vi "Solve1.vi"(8 "Error In":errorcluster, 11 "object in":refnum<class "2022_6.lvclass">) -> (0 "Error Out":errorcluster, 2 "Result":u64, 3 "object out":refnum<class "2022_6.lvclass">)   [LabVIEW 2020, in "2022_6.lvclass"]
uses:
  2022_6.lvclass
  2022_6.lvclass/2022_6.ctl
  5bf5dcff-f428-4ee2-9bdf-71b01ce05b8f.vi
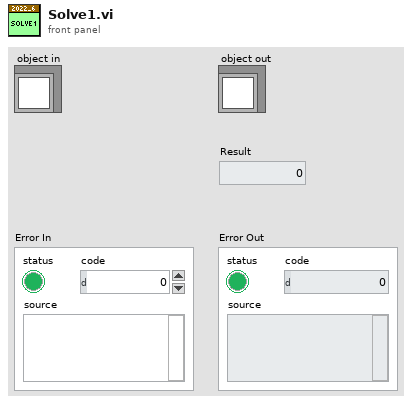
[diagram p1: front panel]
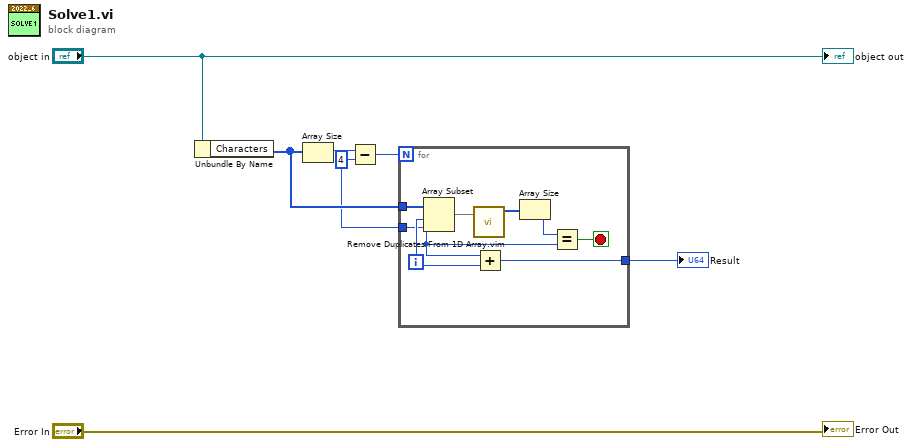
[diagram p0: block diagram]
diagram:
  w2 = 4 ("y")
  n1 = Unbundle By Name("object in") -> ("Characters"=w3:u8[])
  n2 = Array Size(array=w3) -> (size(s)=w5:i32)
  n3 = Subtract(x=w5, y=w2) -> (x-y=w4:i32)
  n4 = for {
    N: w4 -> [_]
    tunnel: w3 -> [w15]
    tunnel: w2 -> [w9]
    tunnel: [w8] -> w1
    i -> [w10]
    stop <- w11 stop-if-true
    n5 = Array Subset(array=w15, index=w10, length=w9) -> (w14:u8[])
    n6 = call "Remove Duplicates From 1D Array.vim"("array"=w14) -> ("array with duplicates removed"=w13:u8[])  [unwired: 10 in]
    n7 = Add(x=w9, y=w10) -> (x+y=w8:i32)
    n8 = Array Size(array=w13) -> (size(s)=w12:i32)
    n9 = Equal?(x=w12, y=w9) -> (x = y?=w11:bool)
  }
  "Result" <- w1
  "Error Out" <- "Error In"
  "object out" <- "object in"
